vi "LSCI332ReadHeater.vi"(0 "VISA Rsrc":refnum<visa-resource-name>="GPIB0::12::INSTR", 5 "Résistance":u16=50, 11 "error in":errorcluster) -> (4 "Puissance(W)":dbl, 6 "Puissance(%)":dbl, 8 "Échelle":u16, 15 "error out":errorcluster)   [LabVIEW 2019]
doc: "Ce Vi interroge l'instrument sur l'échelle de chauffage en watt et le pourcentage de chauffage actuel et retourne une puissance de chauffage en Watts"
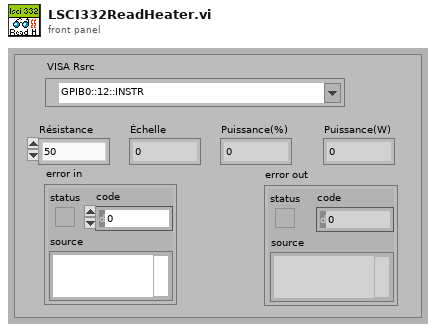
[diagram p1: front panel]
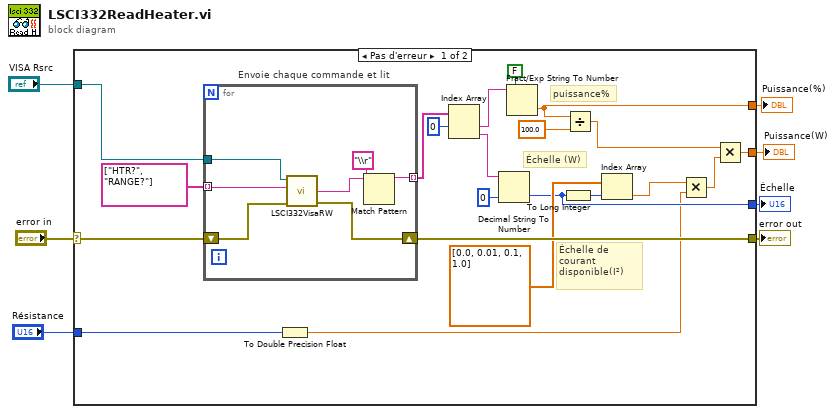
[diagram p0: block diagram]
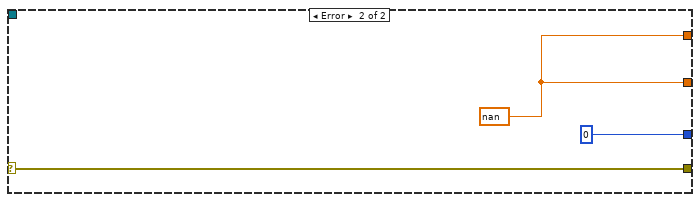
[diagram p2: hidden frame]
diagram:
  n1 = case shown="Pas d'erreur" "error in" {
    selector: "error in" -> [w26 w38]
    tunnel: [w28 w38] -> w7
    tunnel: "VISA Rsrc" -> [w27 _]
    tunnel: [w18 w37] -> w4
    tunnel: [w15 w37] -> w3
    tunnel: [w16 u16 0] -> w2
    tunnel: "Résistance" -> [w11 _]
    frame No Error {
      # "Échelle (W)"
      # "puissance%"
      # "Échelle de courant disponible(I²)"
      # "Envoie chaque commande et lit"
      n2 = for {
        tunnel: string[] ["HTR?", "RANGE?"] -> [w32] mode=indexing
        shift-right: [w30] -> w28
        shift-left: w26 -> [w31]
        tunnel: w27 -> [w33]
        tunnel: [w34] -> w23 mode=indexing
        n3 = call <userlib>:"LSCI332VisaRW.vi"("error in (no error)"=w31, "ChaineCom"=w32, "VISA Rsrc"=w33) -> ("error out"=w30:errorcluster, "ChaineRep"=w29:string)  [unwired: 4 in, 2 out]
        n4 = Match Pattern(string=w29, regular expression="\\r") -> (before substring=w34:string)  [unwired: 1 in, 3 out]
      }
      n5 = To Double Precision Float(number=w11) -> (double precision float=w10:dbl)
      n6 = Index Array(array=w23, index #1=0 ("index")) -> (element #1=w21:string, element #2=w20:string)  [unwired: 1 in]
      n7 = Decimal String To Number(string=w20, default (0L)=u16 0 ("default (0 I32)")) -> (number=w16:u16)  [unwired: 1 in, 1 out]
      n8 = Fract/Exp String To Number(use system decimal point (T)=FALSE, string=w21) -> (number=w15:dbl)  [unwired: 2 in, 1 out]
      n9 = To Long Integer(number=w16) -> (32bit integer=w13:i32)
      n10 = Divide(x=w15, y=100.0) -> (x/y=w9:dbl)
      n11 = Index Array(array=dbl[] [0.0, 0.01, 0.1, 1.0], index=w13) -> (element=w12:dbl)
      n12 = Multiply(x=w12, y=w10) -> (x*y=w8:dbl)
      n13 = Multiply(x=w9, y=w8) -> (x*y=w18:dbl)
    }
    frame Error {
      w37 = nan
    }
  }
  "error out" <- w7
  "Puissance(W)" <- w4
  "Puissance(%)" <- w3
  "Échelle" <- w2
